vi "Test PID.vi"() -> ()   [LabVIEW 2020]
uses:
  IG PID/Parameters.ctl
  IG PID/Output Range.ctl
  IG PID/State.ctl
  IG PID/PID/PID.lvclass
  IG PID/IG PID.lvlib
panel:
  out "Terms":T1
  in  "Reset":bool
  in  "SP":dbl(slide)=137.8590078328982 scale=100.0..140.0
  in  "PV":dbl(slide)=70.49608355091384 scale=100.0..140.0
  out "Chart":T2(graph)
  in  "dT (Auto)":dbl
  in  "Output Range":T3={"Min"=-50.0, "Max"=50.0}
  in  "Parameters":T4={"P Band"=10.0, "I Gain"=0.5, "D Gain"=0.1, "F Gain"=0.0}
  # "Abort to stop"
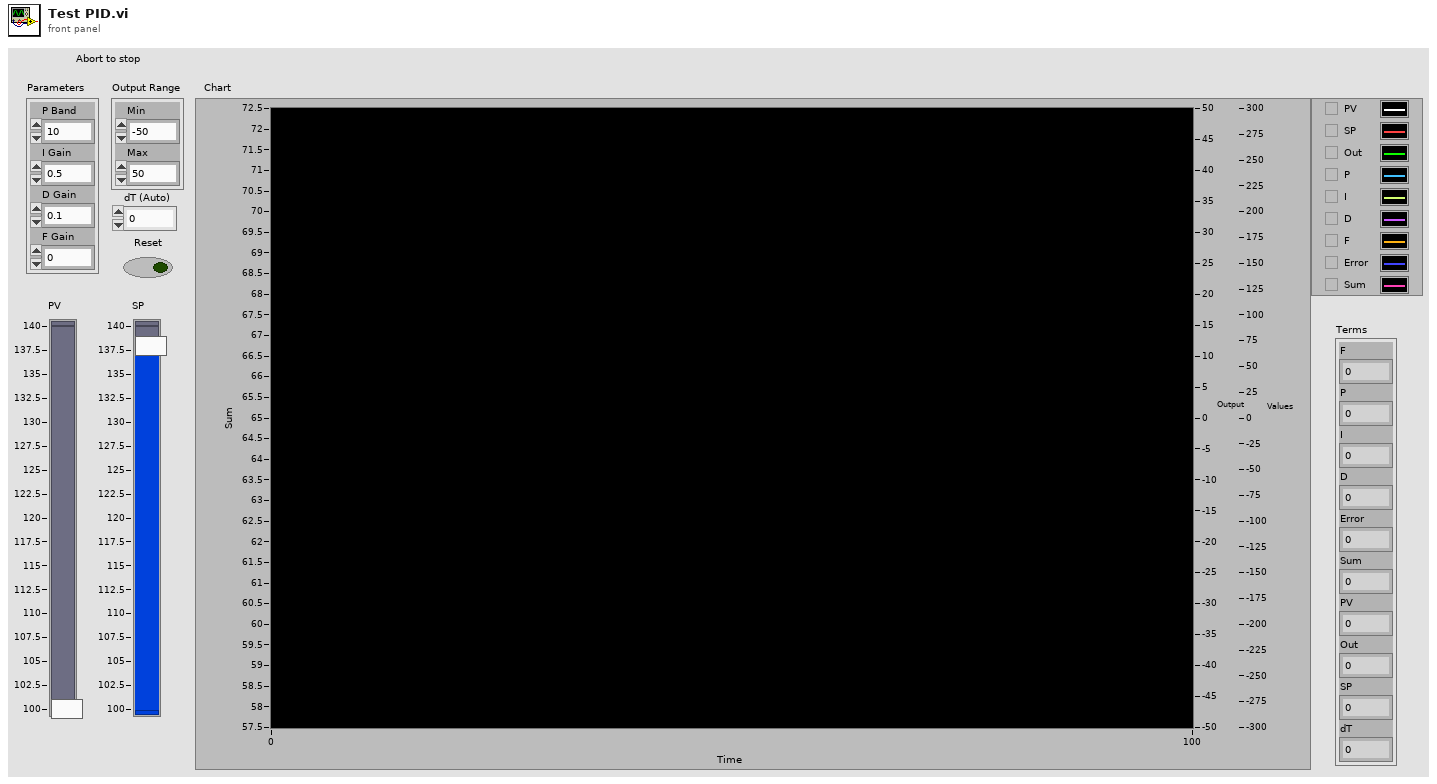
[diagram p1: front panel]
types:
  T1 = typedef "IG PID.lvlib/State.ctl" = cluster{"F":dbl, "P":dbl, "I":dbl, "D":dbl, "Error":dbl, "Sum":dbl, "PV":dbl, "Out":dbl, "SP":dbl, "dT":dbl}
  T2 = cluster{"PV":dbl, "SP":dbl, "Output":dbl, "P":dbl, "I":dbl, "D":dbl, "F":dbl, "F":dbl, "Sum":dbl}
  T3 = typedef "IG PID.lvlib/Output Range.ctl" = cluster{"Min":dbl, "Max":dbl}
  T4 = typedef "IG PID.lvlib/Parameters.ctl" = cluster{"P Band":dbl, "I Gain":dbl, "D Gain":dbl, "F Gain":dbl}
  T5 = cluster{"PV":dbl, "SP":dbl, "Output":dbl, "P":dbl, "I":dbl, "D":dbl, "F":dbl, "Error":dbl, "Sum":dbl}
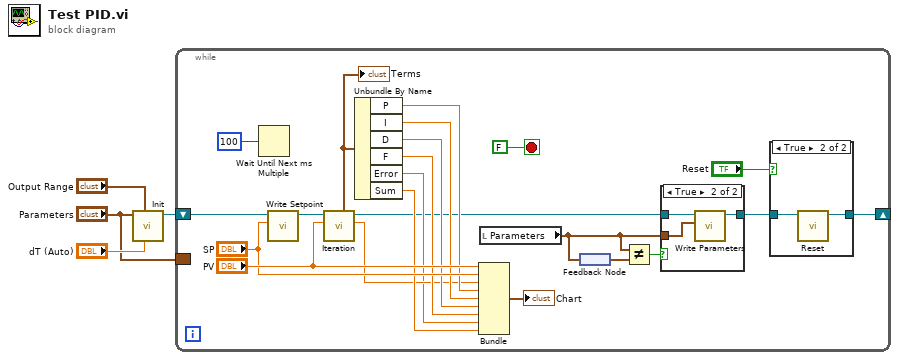
[diagram p0: block diagram]
diagram:
  n1 = call "Init.vi"("dT (Auto)"="dT (Auto)", "Output Range"="Output Range", "Parameters"="Parameters") -> ("PID out"=w2:refnum<class "PID.lvclass">)  [unwired: 7 in, 1 out]
  n2 = while {
    shift-right: [w5] -> _
    shift-left: w2 -> [w26]
    border: "Parameters" -> [_]
    stop <- FALSE stop-if-true
    n3 = Wait Until Next ms Multiple(millisecond multiple=u32 100) -> ()  [unwired: 1 out]
    n4 = call "Write Setpoint.vi"("Setpoint"="SP", "PID in"=w26) -> ("PID out"=w24:refnum<class "PID.lvclass">)  [unwired: 8 in, 1 out]
    n5 = call "Iteration.vi"("Process Value"="PV", "PID in"=w24) -> ("Output"=w13:dbl, "PID out"=w10:refnum<class "PID.lvclass">, "Terms"=w25:T1)  [unwired: 6 in, 1 out]
    "Terms" <- w25
    n6 = Unbundle By Name(w25) -> ("P"=w20:dbl, "I"=w19:dbl, "D"=w18:dbl, "F"=w17:dbl, "Error"=w12:dbl, "Sum"=w16:dbl)
    n7 = Bundle("PV"="PV", "SP"="SP", "Output"=w13, "P"=w20, "I"=w19, "D"=w18, "F"=w17, "Error"=w12, "Sum"=w16) -> (→"Chart":T5)  [unwired: 1 in]
    n8 = local read "Parameters"() -> (w8:T4)
    n9 = feedback #1() -> (w11:T4)
    n10 = feedback-in #1(w8) -> ()
    n11 = Not Equal?(x=w8, y=w11) -> (x != y?=w9:bool)
    n12 = case shown="True" w9 {
      tunnel: w10 -> [w30 w33]
      tunnel: [w30 w31] -> w7
      tunnel: w8 -> [_ w32]
      frame False {
      }
      frame True {
        n13 = call "Write Parameters.vi"("Parameters"=w32, "PID in"=w33) -> ("PID out"=w31:refnum<class "PID.lvclass">)  [unwired: 8 in, 1 out]
      }
    }
    n14 = case shown="True" "Reset" {
      tunnel: w7 -> [w27 w29]
      tunnel: [w27 w28] -> w5
      frame False {
      }
      frame True {
        n15 = call "Reset.vi"("PID in"=w29) -> ("PID out"=w28:refnum<class "PID.lvclass">)  [unwired: 9 in, 1 out]
      }
    }
  }
